vi "Actor API Type.vi"(11 "Actor in":refnum<class "Actor.lvclass">) -> (2 "Actor API Type":refnum<class "Actor API.lvclass">)   [LabVIEW 2022 SP3, in "Artifex.lvlib" / "Actor.lvclass"]
uses:
  Actor.lvclass
  Actor Proxy/Actor API.lvclass
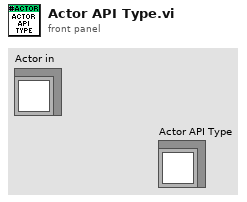
[diagram p1: front panel]
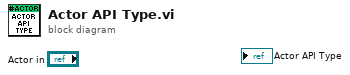
[diagram p0: block diagram]
diagram:
